vi "gds_source.vi"(8 "error in (no error)":errorcluster, 11 "Modulation Parameters In":T1) -> (0 "error out":errorcluster, 2 "Key Bit Sequence":i8[](array[numeric]), 3 "Modulation Parameters Out":T1)   [LabVIEW 2012]
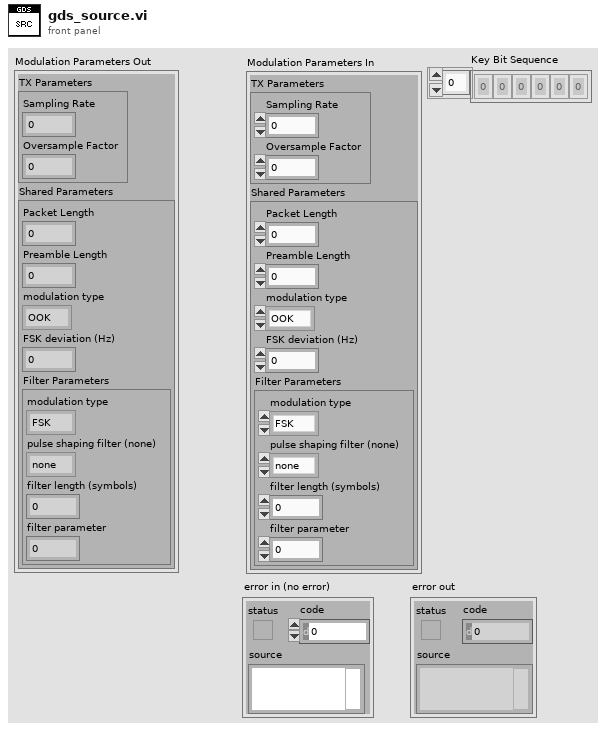
[diagram p1: front panel]
types:
  T1 = cluster{"TX Parameters":cluster{"Sampling Rate":dbl, "Oversample Factor":i32}, "Shared Parameters":cluster{"Packet Length":i32, "Preamble Length":i32, "modulation type":enum16{"OOK", "FSK", "PSK", "QAM", "MSK", "PAM", "ASK", "CPM"}, "FSK deviation (Hz)":dbl, "Filter Parameters":cluster{"modulation type":enum16{"FSK", "PSK", "QAM", "MSK", "PAM", "ASK", "CPM"}, "pulse shaping filter (none)":enum16{"none", "Raised Cosine", "Root Raised Cos", "Gaussian"}, "filter length (symbols)":i32, "filter parameter":dbl}}}
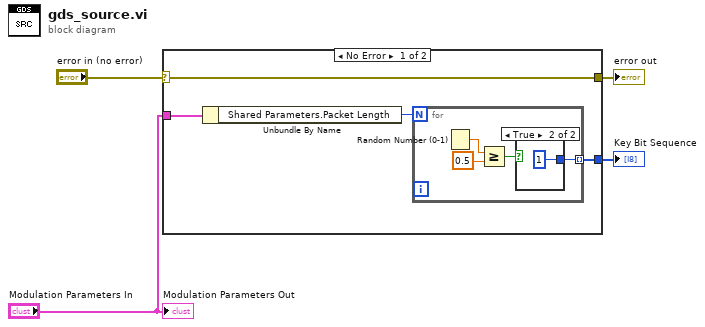
[diagram p0: block diagram]
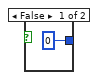
[diagram p2: hidden frame]
diagram:
  n1 = case shown="No Error" "error in (no error)" {
    selector: "error in (no error)" -> [w8 w15]
    tunnel: [w8 w15] -> w3
    tunnel: [w7 _] -> w2
    tunnel: "Modulation Parameters In" -> [w6 _]
    frame No Error {
      n2 = Unbundle By Name(w6) -> ("Shared Parameters.Packet Length"=w5:i32)
      n3 = for {
        N: w5 -> [_]
        tunnel: [w9] -> w7 mode=indexing
        n4 = Random Number (0-1)() -> (number: 0 to 1=w11:dbl)
        n5 = Greater Or Equal?(x=w11, y=0.5) -> (x >= y?=w10:bool)
        n6 = case shown="True" w10 {
          tunnel: [i8 0 i8 1] -> w9
          frame False {
          }
          frame True {
          }
        }
      }
    }
    frame Error {
    }
  }
  "Key Bit Sequence" <- w2
  "error out" <- w3
  "Modulation Parameters Out" <- "Modulation Parameters In"
